vi "Get Http Client Handle.vi"(11 "Refnum in":T1) -> (3 "Refnum out":T1)   [LabVIEW 2023, in "LabVIEW AI Base.lvlib"]
uses:
  LabVIEW AI Base.lvlib
  <vilib>/httpClient/ClientHandle.ctl
  AI Base Globals.vi
  <vilib>/httpClient/LabVIEWHTTPClient.lvlib
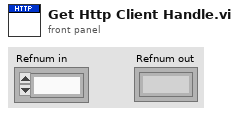
[diagram p1: front panel]
types:
  T1 = typedef "LabVIEWHTTPClient.lvlib/ClientHandle.ctl" = refnum<k1>
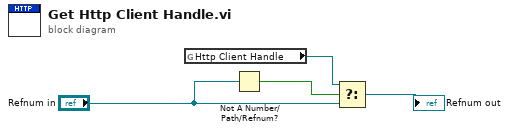
[diagram p0: block diagram]
diagram:
  n1 = global read "AI Base Globals.vi" "Http Client Handle"() -> (w4:T1)
  n2 = Not A Number/Path/Refnum?(number/path/refnum="Refnum in") -> (NaN/Path/Refnum?=w3:bool)
  n3 = Select(t=w4, s=w3, f="Refnum in") -> (s? t:f=→"Refnum out":T1)
